vi "calc std seq values.vi"(8 "error in":errorcluster, 9 "which measurements":string[](array[string])=["average cycle ratio", "std seq counts", "std seq q", "std seq ratio", "std seq norm", "std internal error", "std internal error(%)", "std external error", "std external error(%)", "std error", "ext vs int"], 10 "cycle results labels":string[](array[string]), 11 "std cycle results dbl":dbl[][](array[numeric])) -> (0 "error out":errorcluster, 3 "std seq results":dbl[](array[numeric]))   [LabVIEW 2016]
panel:
  out "subarray":dbl[](array[numeric])
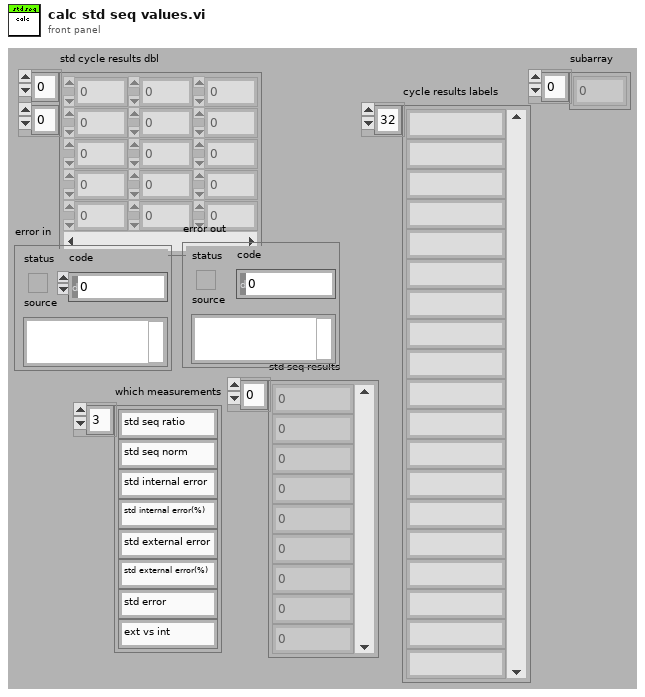
[diagram p1: front panel]
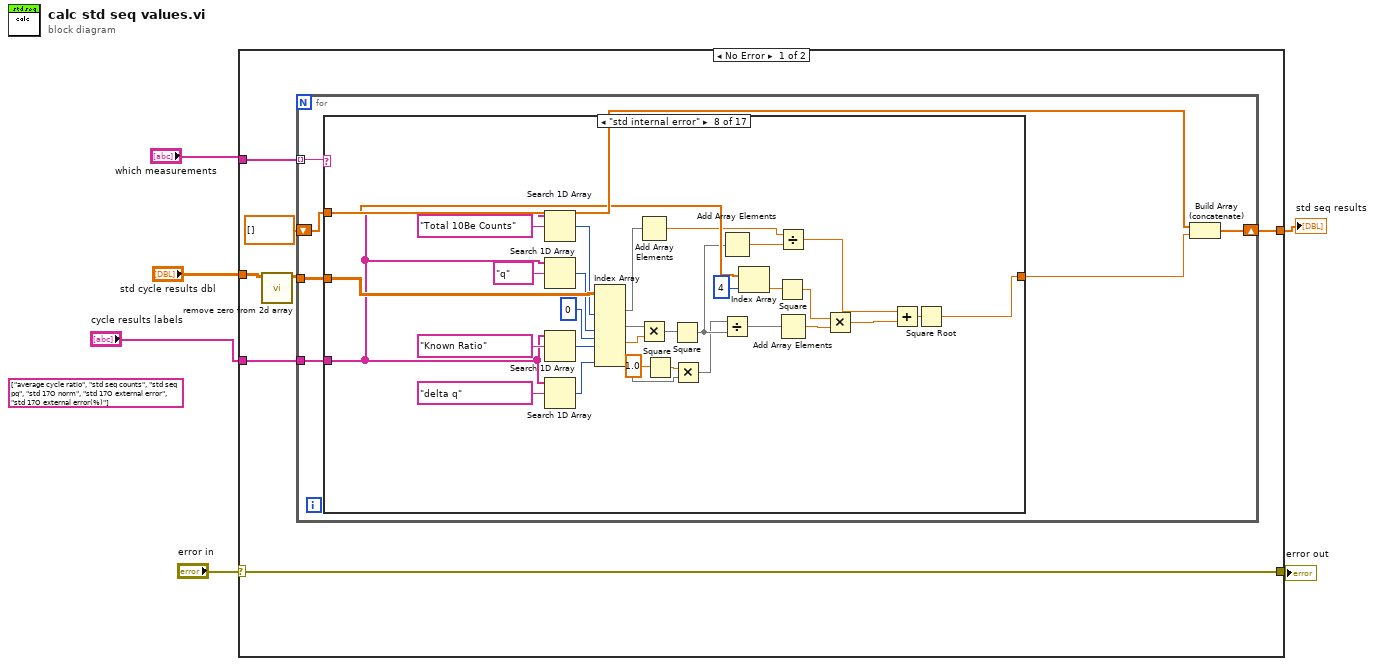
[diagram p0: block diagram]
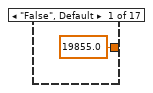
[diagram p2: hidden frame]
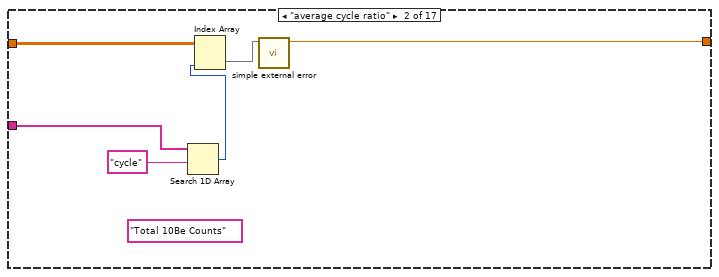
[diagram p3: hidden frame]
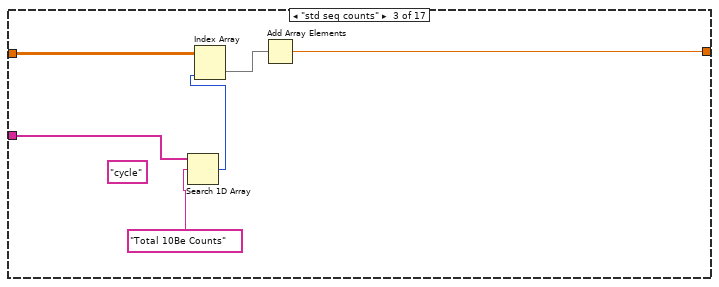
[diagram p4: hidden frame]
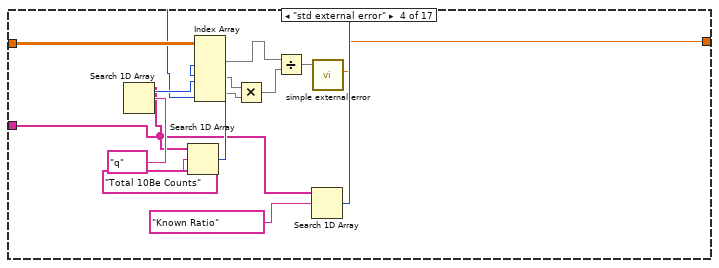
[diagram p5: hidden frame]
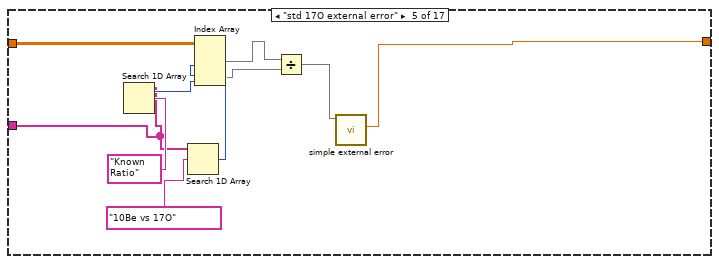
[diagram p6: hidden frame]
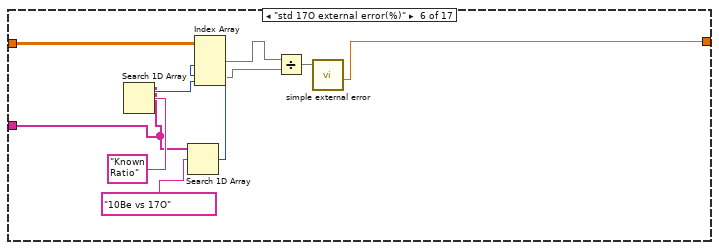
[diagram p7: hidden frame]
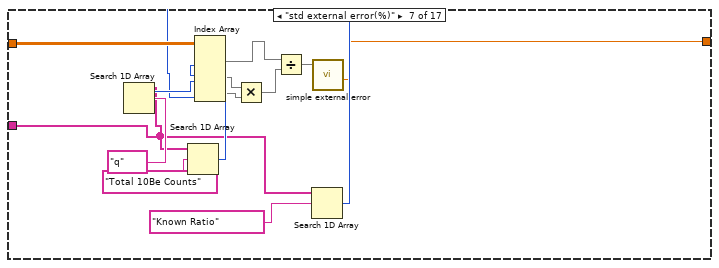
[diagram p8: hidden frame]
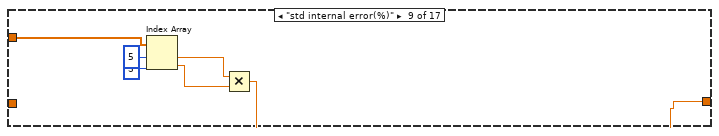
[diagram p9: hidden frame]
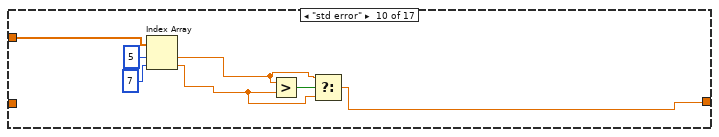
[diagram p10: hidden frame]
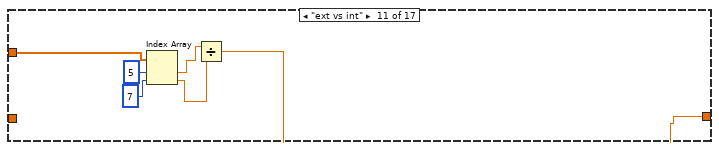
[diagram p11: hidden frame]
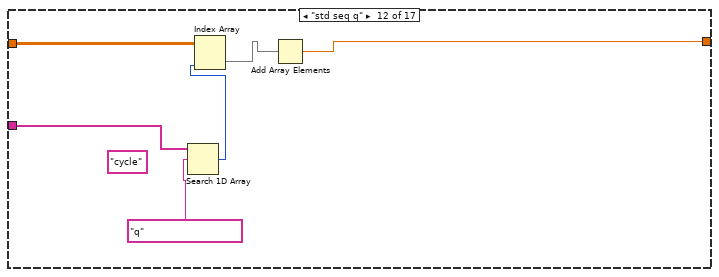
[diagram p12: hidden frame]
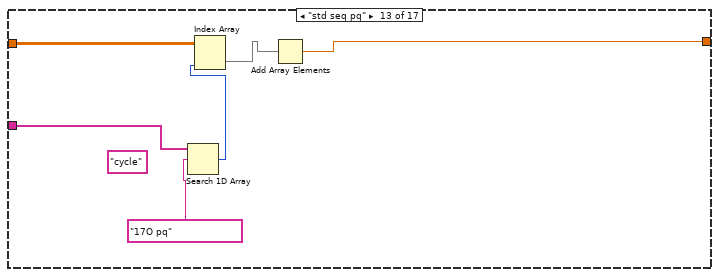
[diagram p13: hidden frame]
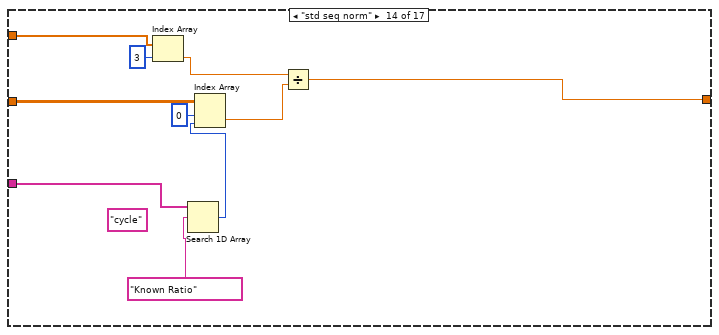
[diagram p14: hidden frame]
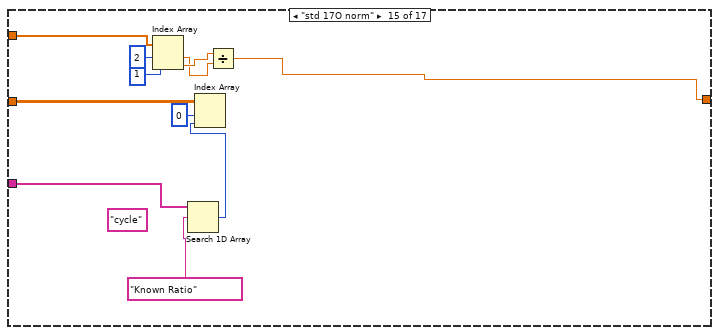
[diagram p15: hidden frame]
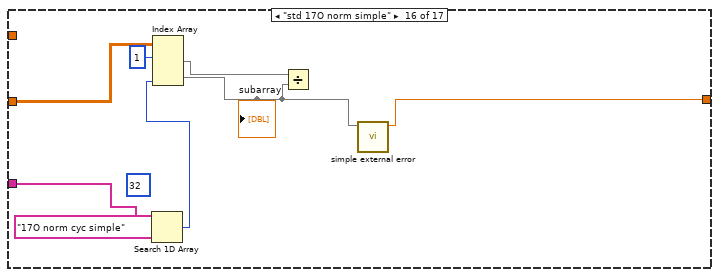
[diagram p16: hidden frame]
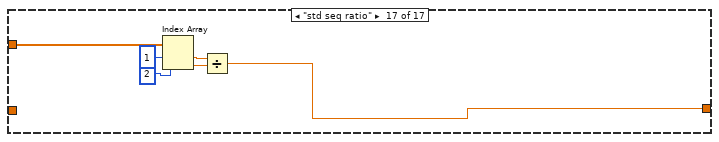
[diagram p17: hidden frame]
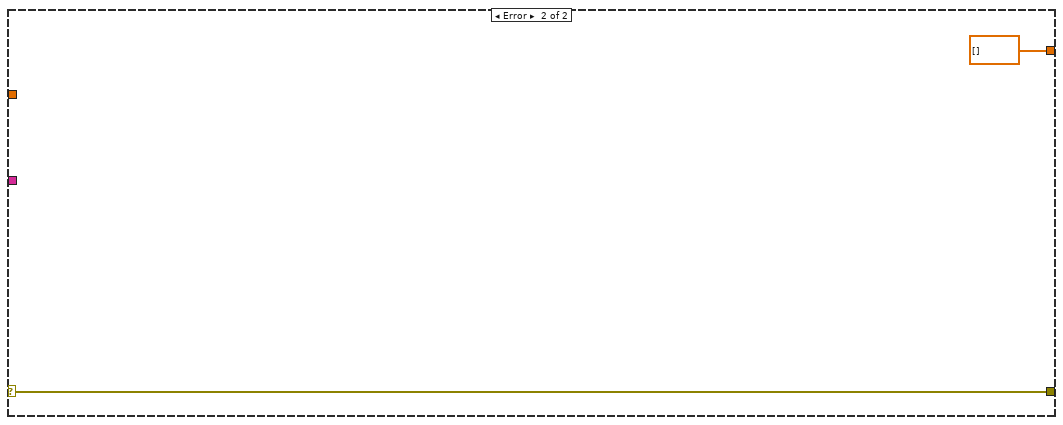
[diagram p18: hidden frame]
diagram:
  (unwired) string[] ["average cycle ratio", "std seq counts", "std seq pq", "std 17O norm", "std 17O external error", "std 17O external error(%)"] ("cycle results labels")
  n1 = case shown="No Error" "error in" {
    selector: "error in" -> [w8 w180]
    tunnel: "which measurements" -> [w7 _]
    tunnel: "std cycle results dbl" -> [w13 _]
    tunnel: "cycle results labels" -> [w12 _]
    tunnel: [w9 dbl[] []] -> w6
    tunnel: [w8 w180] -> w4
    frame No Error {
      n2 = call "remove zero from 2d array.vi"("Cycle data by seq"=w13) -> ("array w/ subset deleted"=w11:dbl[][])  [unwired: 10 in]
      n3 = for {
        tunnel: w11 -> [w18]
        tunnel: w7 -> [w19] mode=indexing
        tunnel: w12 -> [w17]
        shift-right: [w15] -> w9
        shift-left: dbl[] [] -> [w14]
        n4 = case shown="\"std internal error\"" w19 {
          tunnel: w18 -> [_ w24 w31 w46 w56 w66 w80 w112 _ _ _ w136 w142 w152 w163 w170 _]
          tunnel: w17 -> [_ w25 w32 w38 w51 w61 w72 w105 _ _ _ w137 w143 w153 w164 w167 _]
          tunnel: [19855.0 ("Sequence result") w21 w27 w33 w48 w59 w67 w86 w113 w119 w126 w132 w138 w144 w154 w168 w173] -> w16
          tunnel: w14 -> [_ _ _ _ _ _ _ w99 w118 w125 w131 _ _ w147 w159 _ w178]
          frame "False", Default {
          }
          frame "average cycle ratio" {
            (unwired) "Total 10Be Counts" ("element")
            n5 = Search 1D Array(1D array=w25, element="cycle") -> (index of element=w23:i32)  [unwired: 1 in]
            n6 = Index Array(array=w24, index (col)=w23) -> (element=w22:dbl[])  [unwired: 1 in]
            n7 = call "simple external error.vi"("cycle results"=w22) -> ("Sequence result"=w21:dbl)  [unwired: 7 in, 3 out]
          }
          frame "std seq counts" {
            (unwired) "cycle" ("element")
            n8 = Search 1D Array(1D array=w32, element="Total 10Be Counts") -> (index of element=w30:i32)  [unwired: 1 in]
            n9 = Index Array(array=w31, index (col)=w30) -> (element=w28:dbl[])  [unwired: 1 in]
            n10 = Add Array Elements(numeric array=w28) -> (sum=w27:dbl)
          }
          frame "std external error" {
            n11 = Search 1D Array(1D array=w38, element="q") -> (index of element=w42:i32)  [unwired: 1 in]
            n12 = Search 1D Array(1D array=w38, element="Total 10Be Counts") -> (index of element=w45:i32)  [unwired: 1 in]
            n13 = Search 1D Array(1D array=w38, element="Known Ratio") -> (index of element=w37:i32)  [unwired: 1 in]
            n14 = Index Array(array=w46, index (col) #1=w45, index (col) #2=w42, index (col) #3=w37) -> (element #1=w41:dbl[], element #2=w35:dbl[], element #3=w36:dbl[])  [unwired: 3 in]
            n15 = Multiply(x=w35, y=w36) -> (x*y=w34:dbl[])
            n16 = Divide(x=w41, y=w34) -> (x/y=w40:dbl[])
            n17 = call "simple external error.vi"("cycle results"=w40) -> ("External error"=w33:dbl)  [unwired: 7 in, 3 out]
          }
          frame "std 17O external error" {
            n18 = Search 1D Array(1D array=w51, element="Known Ratio") -> (index of element=w52:i32)  [unwired: 1 in]
            n19 = Search 1D Array(1D array=w51, element="10Be vs 17O") -> (index of element=w55:i32)  [unwired: 1 in]
            n20 = Index Array(array=w56, index (col) #1=w55, index (col) #2=w52) -> (element #1=w49:dbl[], element #2=w50:dbl[])  [unwired: 2 in]
            n21 = Divide(x=w49, y=w50) -> (x/y=w47:dbl[])
            n22 = call "simple external error.vi"("cycle results"=w47) -> ("External error"=w48:dbl)  [unwired: 7 in, 3 out]
          }
          frame "std 17O external error(%)" {
            n23 = Search 1D Array(1D array=w61, element="Known Ratio") -> (index of element=w62:i32)  [unwired: 1 in]
            n24 = Search 1D Array(1D array=w61, element="10Be vs 17O") -> (index of element=w65:i32)  [unwired: 1 in]
            n25 = Index Array(array=w66, index (col) #1=w65, index (col) #2=w62) -> (element #1=w58:dbl[], element #2=w60:dbl[])  [unwired: 2 in]
            n26 = Divide(x=w58, y=w60) -> (x/y=w57:dbl[])
            n27 = call "simple external error.vi"("cycle results"=w57) -> ("percent error"=w59:dbl)  [unwired: 7 in, 3 out]
          }
          frame "std external error(%)" {
            n28 = Search 1D Array(1D array=w72, element="q") -> (index of element=w76:i32)  [unwired: 1 in]
            n29 = Search 1D Array(1D array=w72, element="Total 10Be Counts") -> (index of element=w79:i32)  [unwired: 1 in]
            n30 = Search 1D Array(1D array=w72, element="Known Ratio") -> (index of element=w71:i32)  [unwired: 1 in]
            n31 = Index Array(array=w80, index (col) #1=w79, index (col) #2=w76, index (col) #3=w71) -> (element #1=w75:dbl[], element #2=w69:dbl[], element #3=w70:dbl[])  [unwired: 3 in]
            n32 = Multiply(x=w69, y=w70) -> (x*y=w68:dbl[])
            n33 = Divide(x=w75, y=w68) -> (x/y=w74:dbl[])
            n34 = call "simple external error.vi"("cycle results"=w74) -> ("percent error"=w67:dbl)  [unwired: 7 in, 3 out]
          }
          frame "std internal error" {
            n35 = Search 1D Array(1D array=w105, element="Total 10Be Counts") -> (index of element=w111:i32)  [unwired: 1 in]
            n36 = Search 1D Array(1D array=w105, element="q") -> (index of element=w108:i32)  [unwired: 1 in]
            n37 = Search 1D Array(1D array=w105, element="Known Ratio") -> (index of element=w106:i32)  [unwired: 1 in]
            n38 = Search 1D Array(1D array=w105, element="delta q") -> (index of element=w97:i32)  [unwired: 1 in]
            n39 = Index Array(array=w112, index (col) #1=w111, index (col) #2=w108, index (row) #3=0 ("disabled index (row)"), index (col) #3=w106, index (col) #4=w97) -> (element #1=w92:dbl[], element #2=w101:dbl[], element #3=w102:dbl, element #4=w95:dbl[])  [unwired: 3 in]
            n40 = Add Array Elements(numeric array=w92) -> (sum=w90:dbl)
            n41 = Multiply(x=w101, y=w102) -> (x*y=w100:dbl[])
            n42 = Square(x=1.0) -> (x^2=w96:dbl)
            n43 = Square(x=w100) -> (x^2=w84:dbl[])
            n44 = Multiply(x=w96, y=w95) -> (x*y=w83:dbl[])
            n45 = Add Array Elements(numeric array=w84) -> (sum=w91:dbl)
            n46 = Divide(x=w83, y=w84) -> (x/y=w82:dbl[])
            n47 = Index Array(array=w99, index=4) -> (element=w98:dbl)
            n48 = Square(x=w98) -> (x^2=w93:dbl)
            n49 = Divide(x=w90, y=w91) -> (x/y=w89:dbl)
            n50 = Add Array Elements(numeric array=w82) -> (sum=w94:dbl)
            n51 = Multiply(x=w93, y=w94) -> (x*y=w88:dbl)
            n52 = Add(x=w89, y=w88) -> (x+y=w87:dbl)
            n53 = Square Root(x=w87) -> (sqrt(x)=w86:dbl)
          }
          frame "std internal error(%)" {
            n54 = Index Array(array=w118, index #1=5 ("index"), index #2=3 ("index")) -> (element #1=w115:dbl, element #2=w114:dbl)
            n55 = Multiply(x=w115, y=w114) -> (x*y=w113:dbl)
          }
          frame "std error" {
            n56 = Index Array(array=w125, index #1=5 ("index"), index #2=7 ("index")) -> (element #1=w121:dbl, element #2=w120:dbl)
            n57 = Greater?(x=w121, y=w120) -> (0:w122:bool)
            n58 = Select(t=w121, s=w122, f=w120) -> (s? t:f=w119:dbl)
          }
          frame "ext vs int" {
            n59 = Index Array(array=w131, index #1=5 ("index"), index #2=7 ("index")) -> (element #1=w128:dbl, element #2=w127:dbl)
            n60 = Divide(x=w128, y=w127) -> (x/y=w126:dbl)
          }
          frame "std seq q" {
            (unwired) "cycle" ("element")
            n61 = Search 1D Array(1D array=w137, element="q") -> (index of element=w135:i32)  [unwired: 1 in]
            n62 = Index Array(array=w136, index (col)=w135) -> (element=w133:dbl[])  [unwired: 1 in]
            n63 = Add Array Elements(numeric array=w133) -> (sum=w132:dbl)
          }
          frame "std seq pq" {
            (unwired) "cycle" ("element")
            n64 = Search 1D Array(1D array=w143, element="17O pq") -> (index of element=w141:i32)  [unwired: 1 in]
            n65 = Index Array(array=w142, index (col)=w141) -> (element=w139:dbl[])  [unwired: 1 in]
            n66 = Add Array Elements(numeric array=w139) -> (sum=w138:dbl)
          }
          frame "std seq norm" {
            (unwired) "cycle" ("element")
            n67 = Index Array(array=w147, index=3) -> (element=w145:dbl)
            n68 = Search 1D Array(1D array=w153, element="Known Ratio") -> (index of element=w151:i32)  [unwired: 1 in]
            n69 = Index Array(array=w152, index (row)=0 ("disabled index (row)"), index (col)=w151) -> (element=w148:dbl)
            n70 = Divide(x=w145, y=w148) -> (x/y=w144:dbl)
          }
          frame "std 17O norm" {
            (unwired) "cycle" ("element")
            n71 = Index Array(array=w159, index #1=2 ("index"), index #2=1 ("index")) -> (element #1=w155:dbl, element #2=w156:dbl)
            n72 = Search 1D Array(1D array=w164, element="Known Ratio") -> (index of element=w162:i32)  [unwired: 1 in]
            n73 = Index Array(array=w163, index (row)=0 ("disabled index (row)"), index (col)=w162) -> ()  [unwired: 1 out]
            n74 = Divide(x=w156, y=w155) -> (x/y=w154:dbl)
          }
          frame "std 17O norm simple" {
            (unwired) 32 ("index")
            n75 = Search 1D Array(1D array=w167, element="17O norm cyc simple") -> (index of element=w165:i32)  [unwired: 1 in]
            n76 = Index Array(array=w170, index (row) #1=1 ("index"), index (col) #2=w165) -> (element #1=w171:dbl[], element #2=w169:dbl[])  [unwired: 2 in]
            "subarray" <- w169
            n77 = Divide(x=w171, y=w169) -> ()  [unwired: 1 out]
            n78 = call "simple external error.vi"("cycle results"=w169) -> ("Sequence result"=w168:dbl)  [unwired: 7 in, 3 out]
          }
          frame "std seq ratio" {
            n79 = Index Array(array=w178, index #1=1 ("index"), index #2=2 ("index")) -> (element #1=w174:dbl, element #2=w175:dbl)
            n80 = Divide(x=w174, y=w175) -> (x/y=w173:dbl)
          }
        }
        n81 = Build Array (concatenate)(w14, w16) -> (w15:dbl[])
      }
    }
    frame Error {
    }
  }
  "std seq results" <- w6
  "error out" <- w4
